vi "refnumbers.vi"() -> ()   [LabVIEW 2020]
doc: "This global variable contains refnum names. All refnum names are set in Begin."
panel:
  out "Indexer_Beam_Break":string
  out "Intake_Motor_Right":string
  out "Tower_Motor":string
  out "Indexer_Motor":string
  out "Intake_Motor_Left":string
  out "Cowl_Motor":string
  out "Color_Sensor":string
  out "Shooter_Upper":string
  out "Shooter_Lower":string
  out "Turret_Motor":string
  out "Number_of_LEDs":u16
  out "Swerve_2_Shifter":string
  out "Swerve_1_Shifter":string
  out "Swerve_0_Shifter":string
  out "Swerve_3_Shifter":string
  out "Joystick_Manipulator":string
  out "Swerve_3_Azimuth":string
  out "Swerve_2_Azimuth":string
  out "IMU_0":string
  out "Joystick_Driver":string
  out "Compressor":string
  out "Swerve_1_Azimuth":string
  out "Swerve_0_Azimuth":string
  out "Swerve_3_Drive":string
  out "Swerve_2_Drive":string
  out "Swerve_1_Drive":string
  out "Swerve_0_Drive":string
  # "--driver station--"
  # "--drivebase subsystem--"
  # "--shooter subsystem--"
  # "--ball handling subsystem--"
  # "--climber subsystem--"
  # "--miscellaneous--"
  # "--other sensors--"
  # "--turret subsystem--"
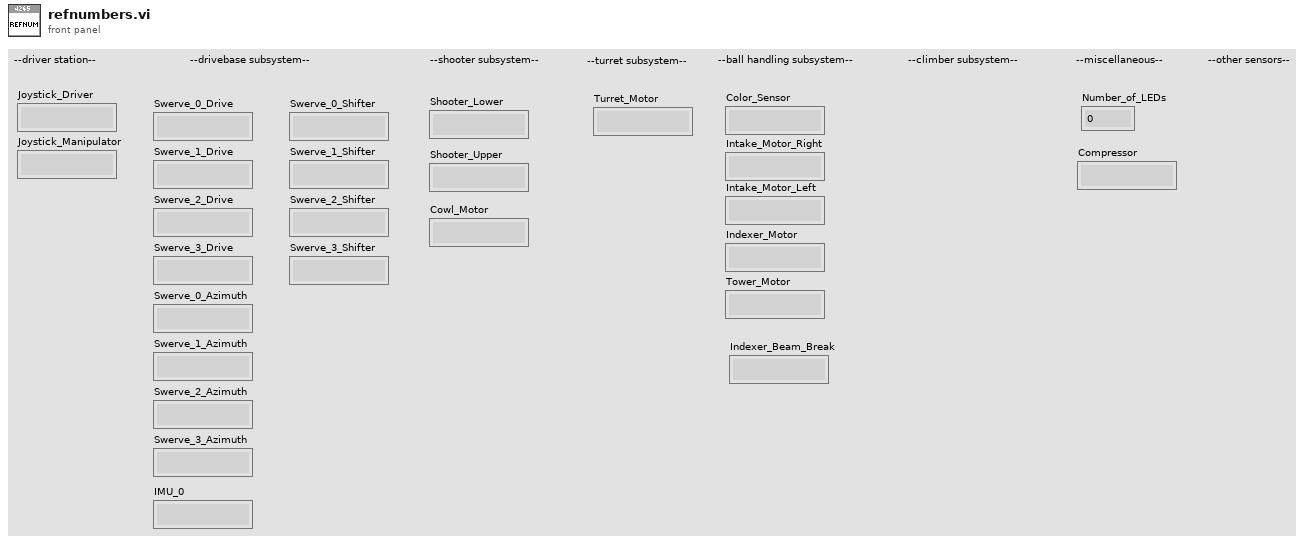
[diagram p1: front panel]
diagram:
